vi "Initialize.vi"(6 "optional":variant, 8 "error in (no error)":errorcluster, 11 "PriorityQueue in":refnum<class "PriorityQueue.lvclass">) -> (0 "error out":errorcluster, 3 "PriorityQueue out":refnum<class "PriorityQueue.lvclass">)   [LabVIEW 2009, in "PriorityQueue.lvclass"]
uses:
  PriorityQueue.lvclass
  BasicSortedList/BasicSortOptions.ctl
  BasicSortedList/BasicSortedList.lvclass
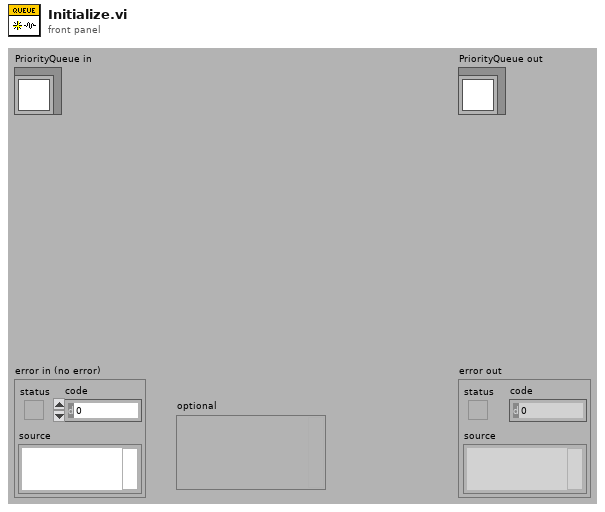
[diagram p1: front panel]
types:
  T1 = typedef "BasicSortedList.lvclass/BasicSortOptions.ctl" = enum16{"Ascending", "Decending"}
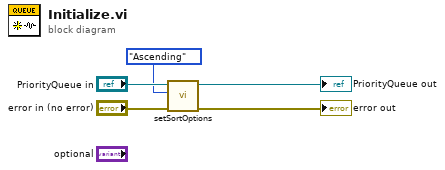
[diagram p0: block diagram]
diagram:
  n1 = call "setSortOptions.vi"("error in (no error)"="error in (no error)", "SortOptions"=BasicSortOptions."Ascending", "BasicSortedList in"="PriorityQueue in") -> ("error out"=→"error out":errorcluster, "BasicSortedList out"=→"PriorityQueue out":refnum<class "PriorityQueue.lvclass">)  [unwired: 7 in]
